vi "ProdaNG.Configurator.LoginGui.vi"() -> (2 "ConnectionString":string, 3 "DB":T1=enum."WPL")   [LabVIEW 2016]
uses:
  ProdaNG.Configurator.DB.ctl
panel:
  in  "User":string="gast"
  in  "Password":string="wabco"
  in  "Database":i32(ring)=2 items=["proda_test", "proda_wpl", "proda_wpl_dev", "proda_wpk"]
  in  "Accept":bool caption="Check"
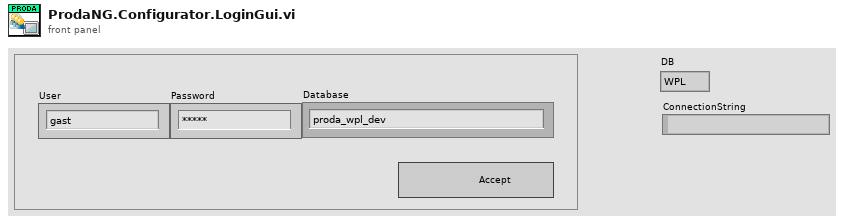
[diagram p1: front panel]
types:
  T1 = typedef "ProdaNG.Configurator.DB.ctl" = enum16{"other", "WPL", "WPK"}
  T2 = enum8{"Enabled", "Disabled", "Disabled and Grayed Out"}
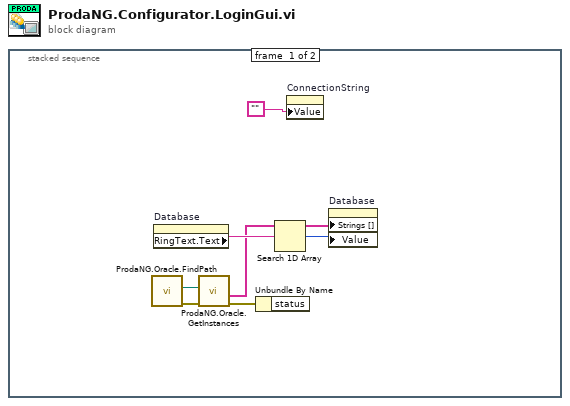
[diagram p0: block diagram]
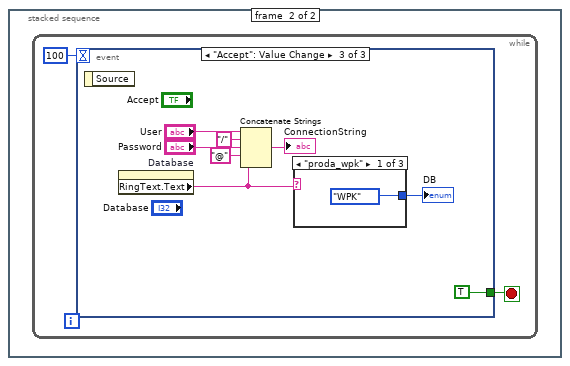
[diagram p2: hidden frame]
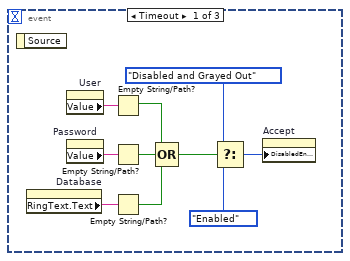
[diagram p3: hidden frame]
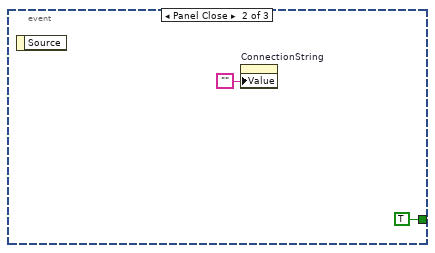
[diagram p4: hidden frame]
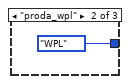
[diagram p5: hidden frame]
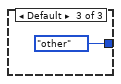
[diagram p6: hidden frame]
diagram:
  n1 = stacked-sequence {
    frame #0 {
      n2 = call "ProdaNG.Oracle.FindPath.vi"() -> ("error out"=w7:errorcluster, "Tnsnames path"=w6:path)  [unwired: 9 in, 1 out]
      n3 = property on="Database" class="Ring (strict)"() -> ("RingText.Text"=w5:string)  [unwired: 2 in, 2 out]
      n4 = call "ProdaNG.Oracle.GetInstances.vi"("error in (no error)"=w7, "Tnsnames path"=w6) -> ("error out"=w3:errorcluster, "Instances Names"=w1:string[])  [unwired: 7 in, 1 out]
      n5 = Unbundle By Name(w3) -> ()  [unwired: 1 out]
      n6 = Search 1D Array(1D array=w1, element=w5) -> (index of element=w4:i32)  [unwired: 1 in]
      n7 = property on="ConnectionString" class="Str"("Value"="") -> ()  [unwired: 2 in, 2 out]
      n8 = property on="Database" class="Ring (strict)"("Strings []"=w1, "Value"=w4) -> ()  [unwired: 2 in, 2 out]
    }
    frame #1 {
      n9 = while {
        stop <- w9 stop-if-true
        n10 = event shown="[2] \"Accept\": Value Change" {
          selector: _ -> [_ _ _]
          dyn-events: _ -> [_ _ _]
          timeout: 100 -> [_ _ _]
          tunnel: [_ TRUE TRUE] -> w9
          event Timeout {
            n11 = event-data() -> ()  [unwired: 1 in, 1 out]
            n12 = property on="Database" class="Ring (strict)"() -> ("RingText.Text"=w10:string)  [unwired: 2 in, 2 out]
            n13 = property on="User" class="Str"() -> ("Value"=w16:string)  [unwired: 2 in, 2 out]
            n14 = property on="Password" class="Str"() -> ("Value"=w19:string)  [unwired: 2 in, 2 out]
            n15 = Empty String/Path?(string/path=w16) -> (empty?=w15:bool)
            n16 = Empty String/Path?(string/path=w19) -> (empty?=w18:bool)
            n17 = Empty String/Path?(string/path=w10) -> (empty?=w17:bool)
            n18 = Compound Arithmetic op=OR(w15, w18, w17) -> (w14:bool)
            n19 = Select(t=T2."Disabled and Grayed Out" ("Disabled"), s=w14, f=T2."Enabled" ("Disabled")) -> (s? t:f=w11:T2)
            n20 = property on="Accept" class="Bool"("DisabledEnum"=w11) -> ()  [unwired: 2 in, 2 out]
          }
          event Panel Close {
            n21 = event-data() -> ()  [unwired: 1 in, 1 out]
            n22 = property on="ConnectionString" class="Str"("Value"="") -> ()  [unwired: 2 in, 2 out]
          }
          event "Accept": Value Change {
            n23 = event-data() -> ()  [unwired: 1 in, 1 out]
            n24 = property on="Database" class="Ring (strict)"() -> ("RingText.Text"=w23:string)  [unwired: 2 in, 2 out]
            n25 = Concatenate Strings("User", "/" ("string"), "Password", "@" ("string"), w23) -> (→"ConnectionString":string)
            n26 = case shown="\"proda_wpk\"" w23 {
              tunnel: [ProdaNG.Configurator.DB."WPK" ("DB") ProdaNG.Configurator.DB."WPL" ("DB") ProdaNG.Configurator.DB."other" ("DB")] -> w22
              frame "proda_wpk" {
              }
              frame "proda_wpl" {
              }
              frame Default {
              }
            }
            "DB" <- w22
          }
        }
      }
    }
  }
